vi "maintenance.vi"() -> ()   [LabVIEW 2019, in "Maintenance.lvlib"]
uses:
  Maintenance.lvlib
panel:
  out "String":string
  out "Tab Control":T1(tab)
  out "Query Verify":errorcluster
  out "Login Log":errorcluster
  out "Login Data Query":errorcluster
  out "General Setting Log":errorcluster
  out "General Setting Database":errorcluster
  out "Threshold Log":errorcluster
  out "Threshold Database":errorcluster
  out "Calibration Method 2 Table":errorcluster
  out "Calibration Method 2 Log":errorcluster
  out "Calibration Method 1 Table":errorcluster
  out "Calibration Method 1 Log":errorcluster
  out "Calibration Method 1 Database":errorcluster
  out "Calibration Setting Log":errorcluster
  out "Calibration Setting Table":errorcluster
  out "Start Application Log":errorcluster
  out "User Table":errorcluster
  out "Log Catalog Table":errorcluster
  out "Search in Log Table":errorcluster
  out "Search in Grading Tables":errorcluster
  out "Save to Excel Report":errorcluster
  out "Print Report":errorcluster
  out "Live View Open VI":errorcluster
  out "Setting Open VI":errorcluster
  out "Report Open VI":errorcluster
  out "Maintenance Open VI":errorcluster
  out "Login Open VI":errorcluster
  out "Logout Log":errorcluster
  out "Graphes Open VI":errorcluster
  out "Shutdown Application Log":errorcluster
  out "Restart Application Log":errorcluster
  out "Close Application Log":errorcluster
  out "Python Close Session":errorcluster
  out "Python Open Session":errorcluster
  out "Python Session out Disc 26":errorcluster
  out "IMAQdx Grab Disc 26":errorcluster
  out "Proc. Calibration Database Disc 26":errorcluster
  out "Python Session in Disc 26":errorcluster
  out "Processing Calibration Disc 26":errorcluster
  out "Speed Signal Log Disc 26":errorcluster
  out "Threshold Calibration Log Disc 26":errorcluster
  out "Main Grading Database Disc 26":errorcluster
  out "Grading Database Disc 26":errorcluster
  out "Pixel to mm Disc 26":errorcluster
  out "Draw Circule Disc 26":errorcluster
  out "IMAQ Copy Disc 26":errorcluster
  out "Log 10001~40002 Disc 26":errorcluster
  out "Image in Disc 26":errorcluster
  out "Image out Disc 26":errorcluster
  out "Python Session out Disc 27":errorcluster
  out "IMAQdx Grab Disc 27":errorcluster
  out "Proc. Calibration Database Disc 27":errorcluster
  out "Python Session in Disc 27":errorcluster
  out "Processing Calibration Disc 27":errorcluster
  out "Speed Signal Log Disc 27":errorcluster
  out "Threshold Calibration Log Disc 27":errorcluster
  out "Main Grading Database Disc 27":errorcluster
  out "Grading Database Disc 27":errorcluster
  out "Pixel to mm Disc 27":errorcluster
  out "Draw Circule Disc 27":errorcluster
  out "IMAQ Copy Disc 27":errorcluster
  out "Image in Disc 27":errorcluster
  out "Image out Disc 27":errorcluster
  out "Log 10001~40002 Disc 27":errorcluster
  out "Python Session out Disc 28":errorcluster
  out "IMAQdx Grab Disc 28":errorcluster
  out "Proc. Calibration Database Disc 28":errorcluster
  out "Python Session in Disc 28":errorcluster
  out "Processing Calibration Disc 28":errorcluster
  out "Speed Signal Log Disc 28":errorcluster
  out "Threshold Calibration Log Disc 28":errorcluster
  out "Main Grading Database Disc 28":errorcluster
  out "Grading Database Disc 28":errorcluster
  out "Pixel to mm Disc 28":errorcluster
  out "Draw Circule Disc 28":errorcluster
  out "IMAQ Copy Disc 28":errorcluster
  out "Image in Disc 28":errorcluster
  out "Image out Disc 28":errorcluster
  out "Log 10001~40002 Disc 28":errorcluster
  out "Python Session out Disc 29":errorcluster
  out "IMAQdx Grab Disc 29":errorcluster
  out "Proc. Calibration Database Disc 29":errorcluster
  out "Python Session in Disc 29":errorcluster
  out "Processing Calibration Disc 29":errorcluster
  out "Speed Signal Log Disc 29":errorcluster
  out "Threshold Calibration Log Disc 29":errorcluster
  out "Main Grading Database Disc 29":errorcluster
  out "Grading Database Disc 29":errorcluster
  out "Pixel to mm Disc 29":errorcluster
  out "Draw Circule Disc 29":errorcluster
  out "IMAQ Copy Disc 29":errorcluster
  out "Image in Disc 29":errorcluster
  out "Image out Disc 29":errorcluster
  out "Log 10001~40002 Disc 29":errorcluster
  out "Python Session out Disc 30":errorcluster
  out "IMAQdx Grab Disc 30":errorcluster
  out "Proc. Calibration Database Disc 30":errorcluster
  out "Python Session in Disc 30":errorcluster
  out "Processing Calibration Disc 30":errorcluster
  out "Speed Signal Log Disc 30":errorcluster
  out "Threshold Calibration Log Disc 30":errorcluster
  out "Main Grading Database Disc 30":errorcluster
  out "Grading Database Disc 30":errorcluster
  out "Pixel to mm Disc 30":errorcluster
  out "Draw Circule Disc 30":errorcluster
  out "IMAQ Copy Disc 30":errorcluster
  out "Image in Disc 30":errorcluster
  out "Image out Disc 30":errorcluster
  out "Log 10001~40002 Disc 30":errorcluster
  in  "Close":bool
  in  "General":bool
  in  "Disc 30":bool
  in  "Disc 29":bool
  in  "Disc 28":bool
  in  "Disc 27":bool
  in  "Disc 26":bool
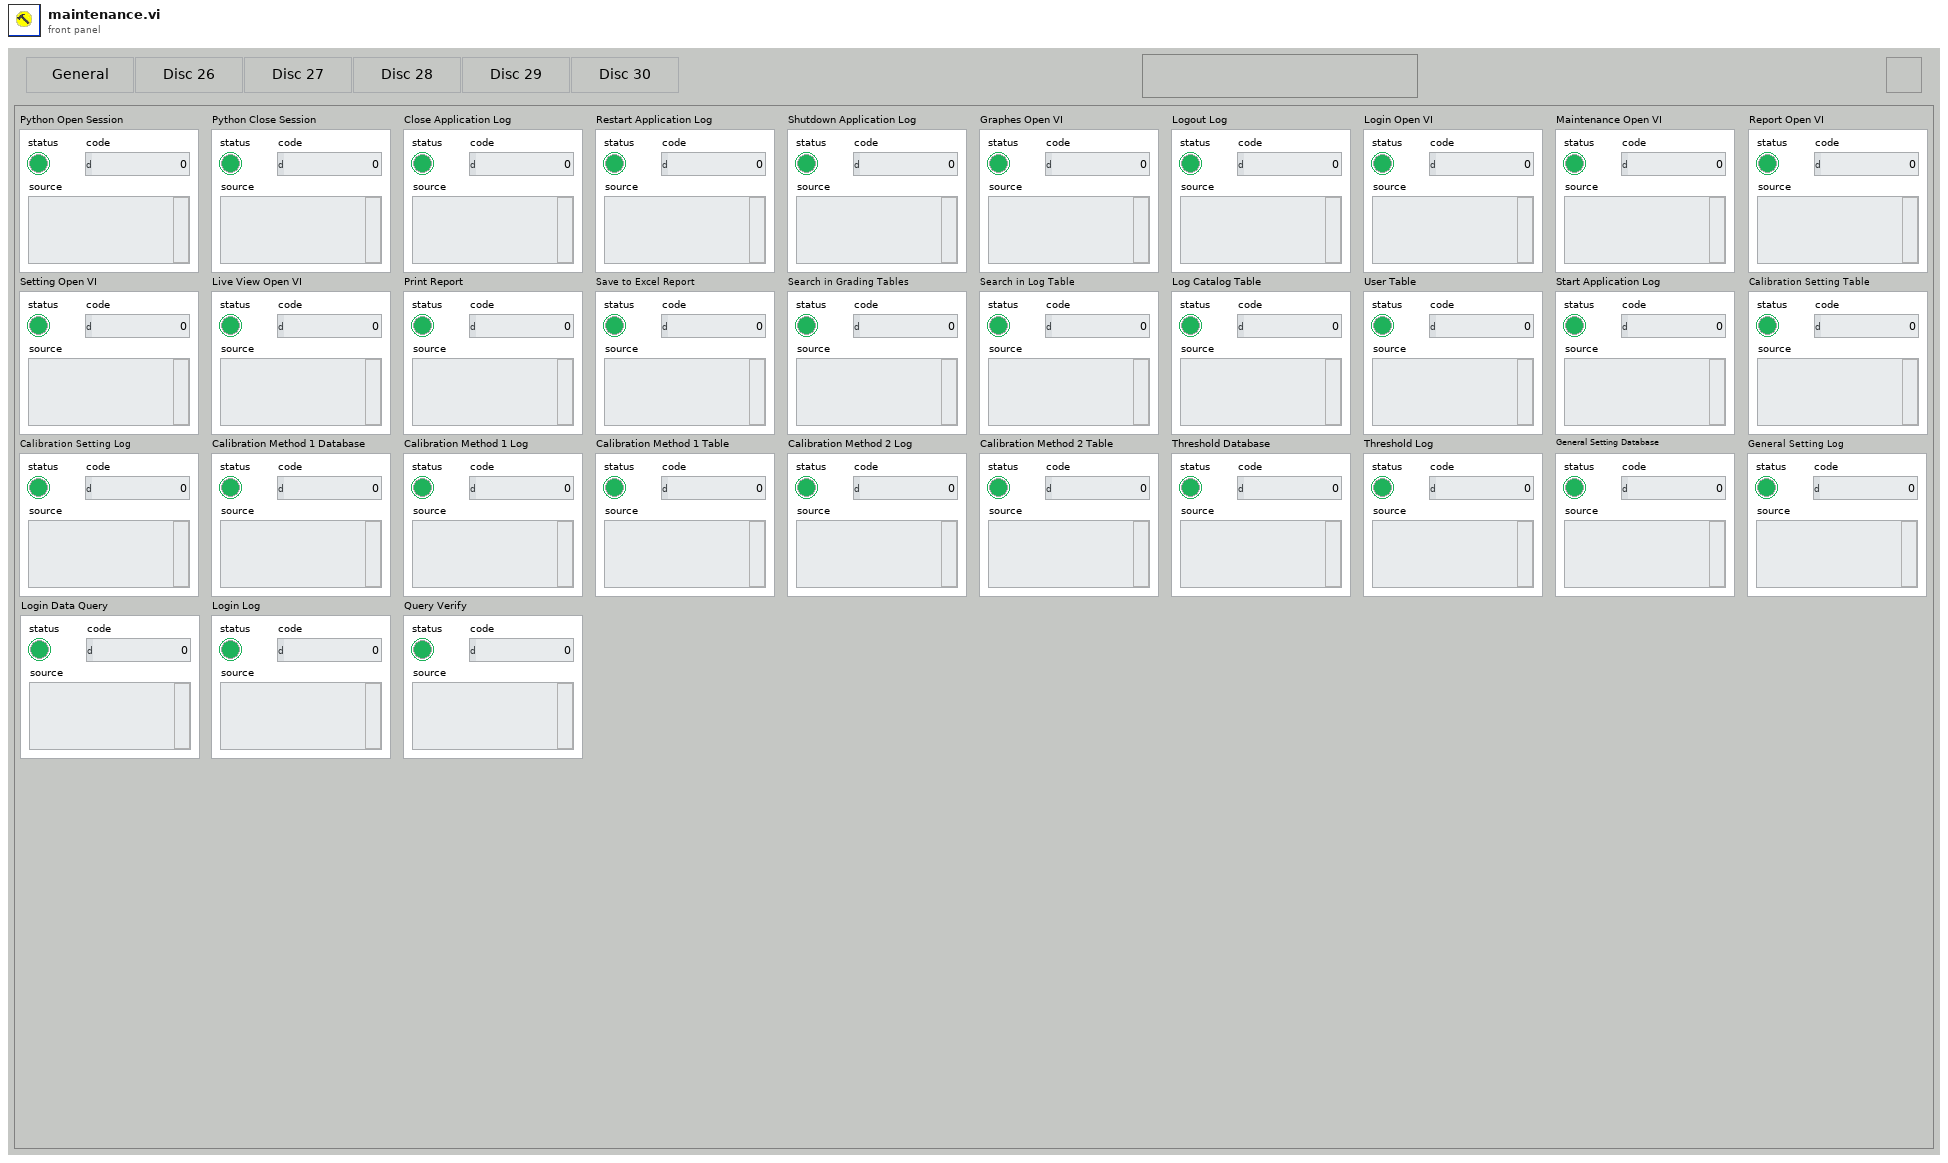
[diagram p1: front panel]
types:
  T1 = enum32{"General", "Disc 26", "Disc 27", "Disc 28", "Disc 29", "Disc 30"}
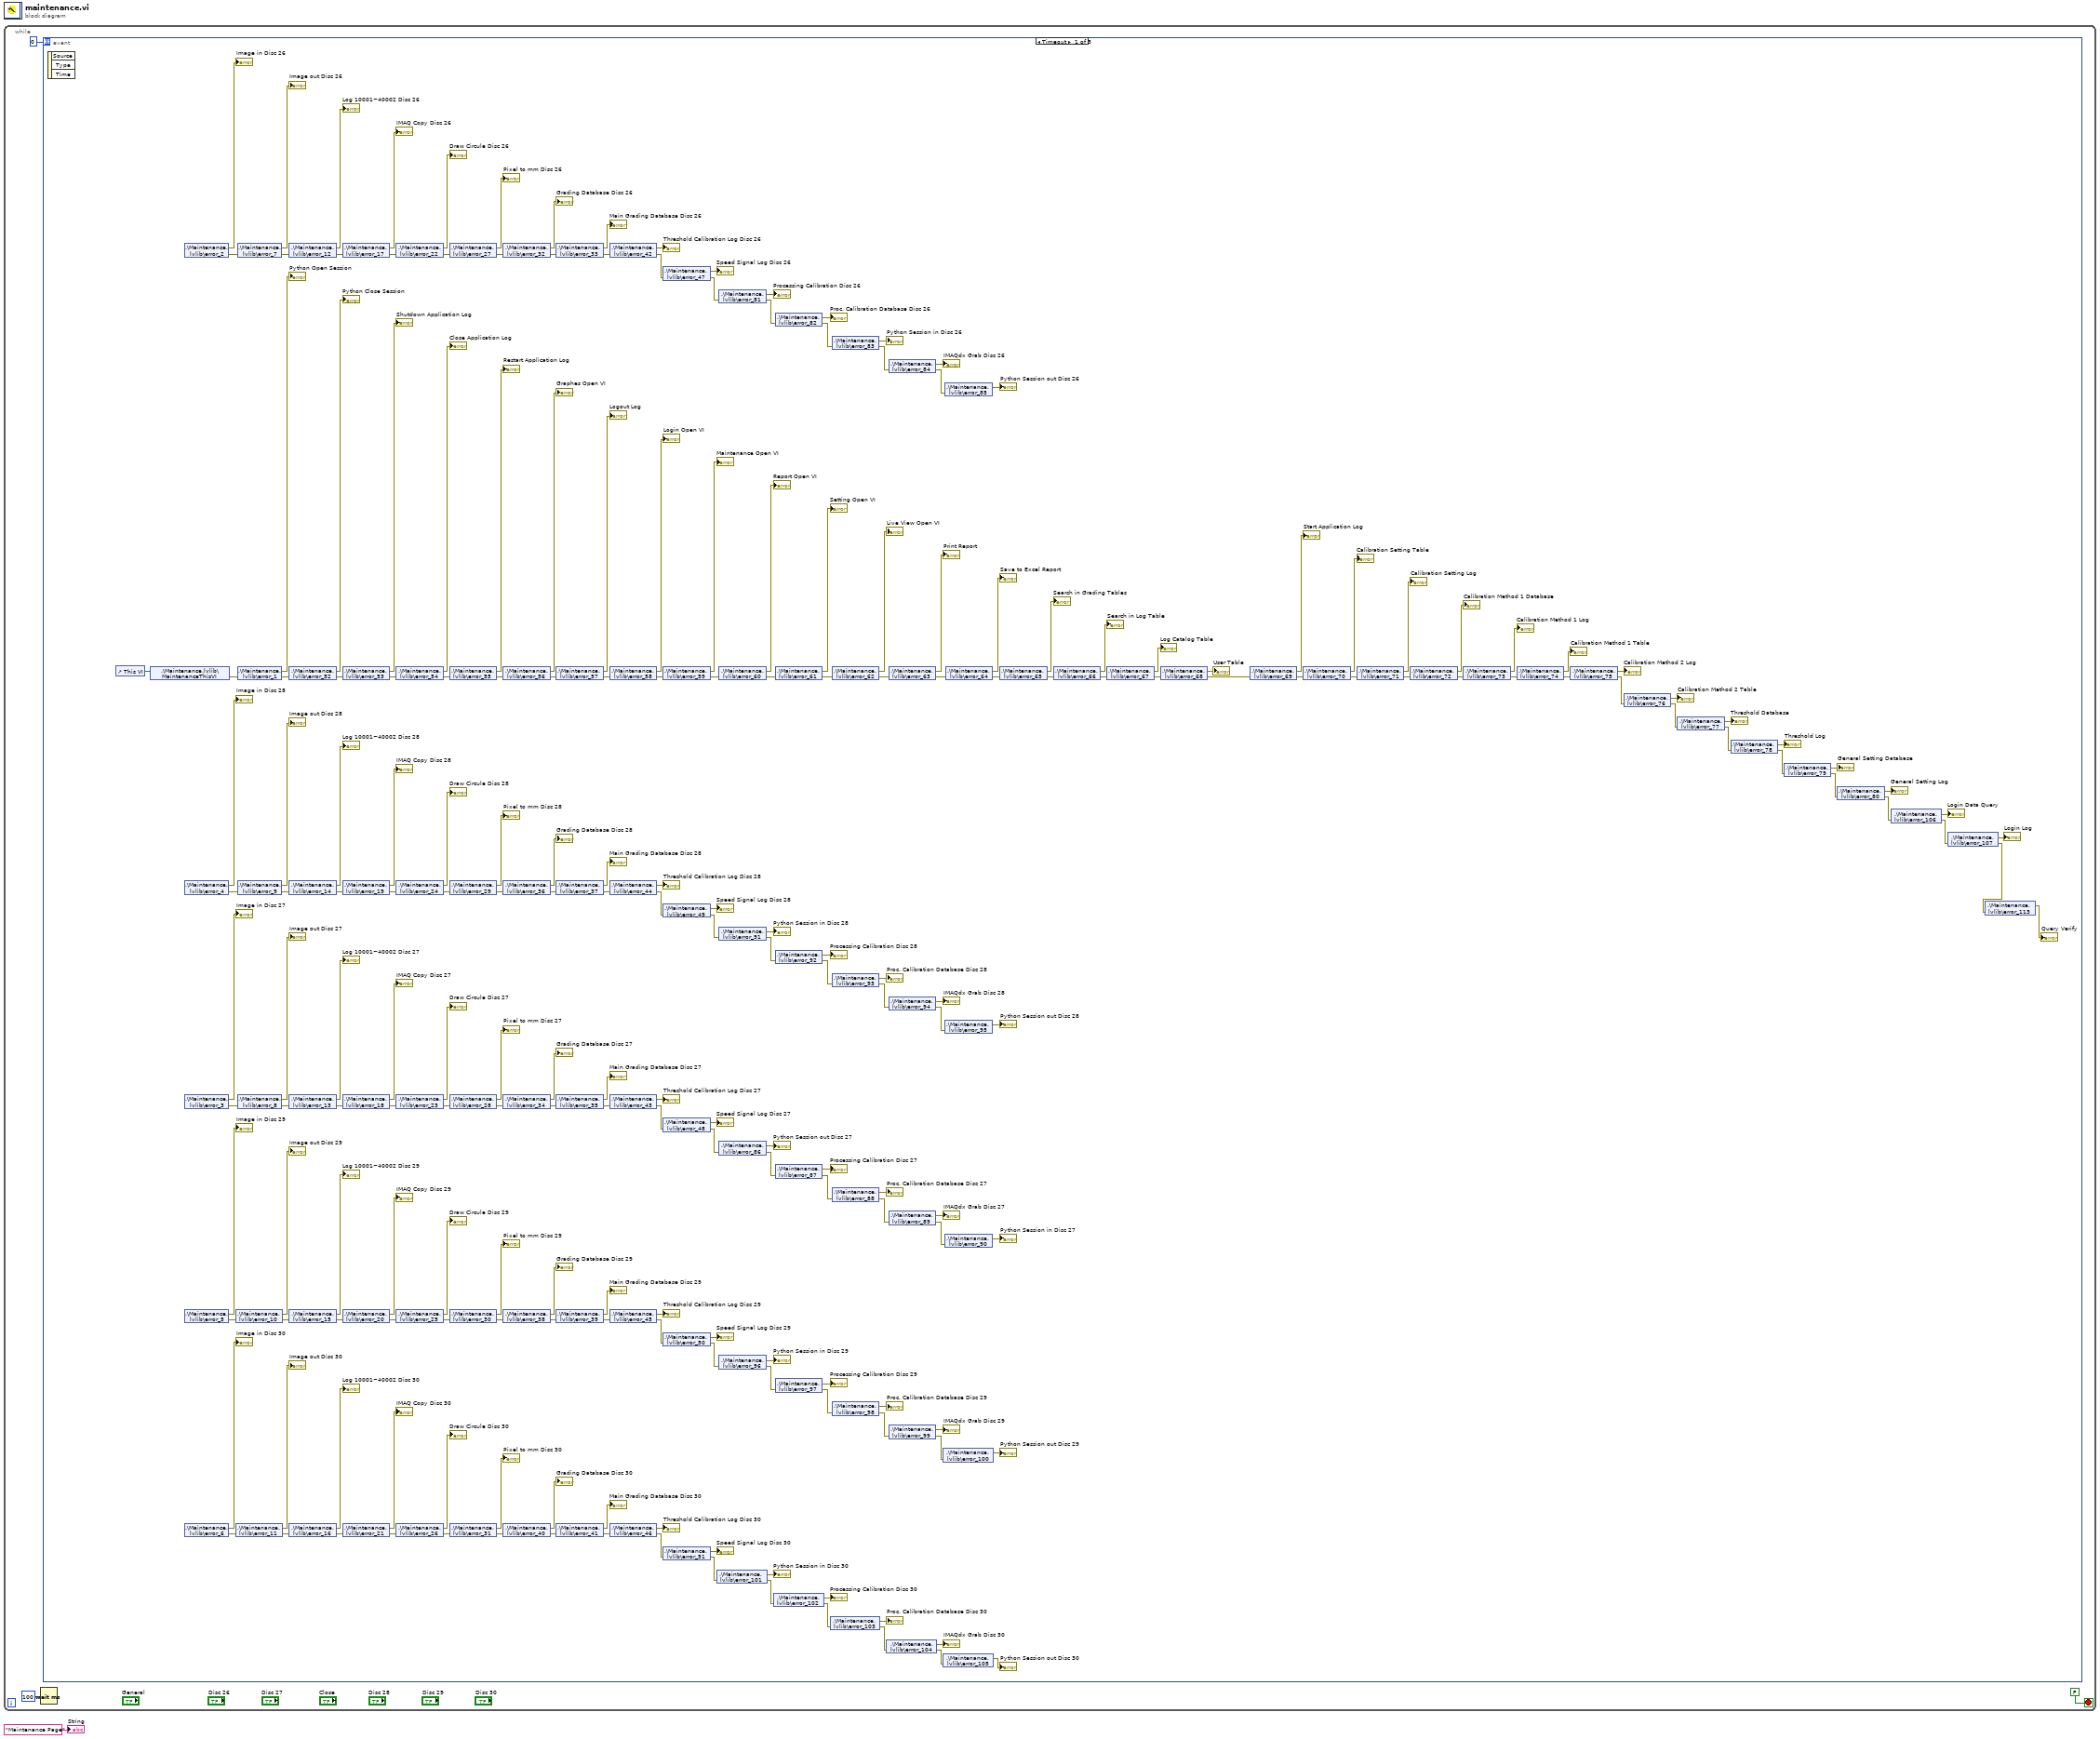
[diagram p0: block diagram]
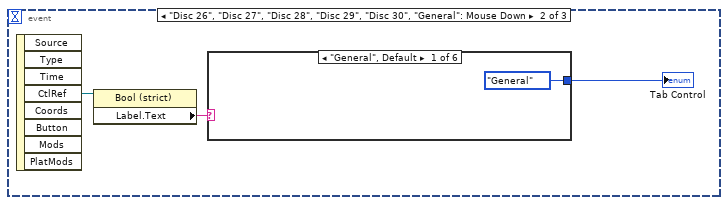
[diagram p2: hidden frame]
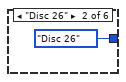
[diagram p3: hidden frame]
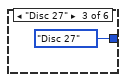
[diagram p4: hidden frame]
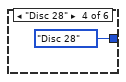
[diagram p5: hidden frame]
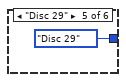
[diagram p6: hidden frame]
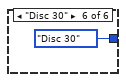
[diagram p7: hidden frame]
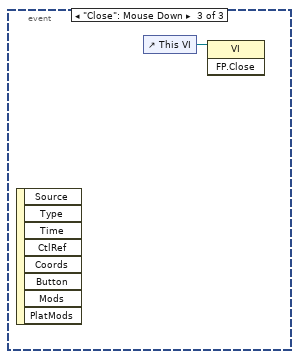
[diagram p8: hidden frame]
diagram:
  n1 = while {
    stop <- FALSE stop-if-true
    n2 = Wait (ms)(milliseconds to wait=u32 100) -> ()  [unwired: 1 out]
    n3 = event shown="[0] Timeout" {
      selector: _ -> [_ _ _]
      dyn-events: _ -> [_ _ _]
      timeout: 0 -> [_ _ _]
      event Timeout {
        n4 = event-data() -> ()  [unwired: 1 in, 3 out]
        n5 = control-ref of="This VI"() -> (w205:refnum<vi>)
        n6 = shared-variable ".\\Maintenance.lvlib\\MaintenanceThisVI"(w205) -> (error out=w189:errorcluster)  [unwired: 1 in]
        n7 = shared-variable ".\\Maintenance.lvlib\\error_2"() -> (→"Image in Disc 26":errorcluster, error out=w198:errorcluster)  [unwired: 1 in]
        n8 = shared-variable ".\\Maintenance.lvlib\\error_4"() -> (→"Image in Disc 28":errorcluster, error out=w199:errorcluster)  [unwired: 1 in]
        n9 = shared-variable ".\\Maintenance.lvlib\\error_3"() -> (→"Image in Disc 27":errorcluster, error out=w194:errorcluster)  [unwired: 1 in]
        n10 = shared-variable ".\\Maintenance.lvlib\\error_5"() -> (→"Image in Disc 29":errorcluster, error out=w195:errorcluster)  [unwired: 1 in]
        n11 = shared-variable ".\\Maintenance.lvlib\\error_6"() -> (→"Image in Disc 30":errorcluster, error out=w193:errorcluster)  [unwired: 1 in]
        n12 = shared-variable ".\\Maintenance.lvlib\\error_10"(error in=w195) -> (→"Image out Disc 29":errorcluster, error out=w190:errorcluster)
        n13 = shared-variable ".\\Maintenance.lvlib\\error_11"(error in=w193) -> (→"Image out Disc 30":errorcluster, error out=w192:errorcluster)
        n14 = shared-variable ".\\Maintenance.lvlib\\error_7"(error in=w198) -> (→"Image out Disc 26":errorcluster, error out=w197:errorcluster)
        n15 = shared-variable ".\\Maintenance.lvlib\\error_1"(error in=w189) -> (→"Python Open Session":errorcluster, error out=w127:errorcluster)
        n16 = shared-variable ".\\Maintenance.lvlib\\error_9"(error in=w199) -> (→"Image out Disc 28":errorcluster, error out=w196:errorcluster)
        n17 = shared-variable ".\\Maintenance.lvlib\\error_8"(error in=w194) -> (→"Image out Disc 27":errorcluster, error out=w191:errorcluster)
        n18 = shared-variable ".\\Maintenance.lvlib\\error_12"(error in=w197) -> (→"Log 10001~40002 Disc 26":errorcluster, error out=w187:errorcluster)
        n19 = shared-variable ".\\Maintenance.lvlib\\error_52"(error in=w127) -> (→"Python Close Session":errorcluster, error out=w111:errorcluster)
        n20 = shared-variable ".\\Maintenance.lvlib\\error_14"(error in=w196) -> (→"Log 10001~40002 Disc 28":errorcluster, error out=w184:errorcluster)
        n21 = shared-variable ".\\Maintenance.lvlib\\error_13"(error in=w191) -> (→"Log 10001~40002 Disc 27":errorcluster, error out=w185:errorcluster)
        n22 = shared-variable ".\\Maintenance.lvlib\\error_15"(error in=w190) -> (→"Log 10001~40002 Disc 29":errorcluster, error out=w181:errorcluster)
        n23 = shared-variable ".\\Maintenance.lvlib\\error_16"(error in=w192) -> (→"Log 10001~40002 Disc 30":errorcluster, error out=w179:errorcluster)
        n24 = shared-variable ".\\Maintenance.lvlib\\error_17"(error in=w187) -> (→"IMAQ Copy Disc 26":errorcluster, error out=w169:errorcluster)
        n25 = shared-variable ".\\Maintenance.lvlib\\error_53"(error in=w111) -> (→"Shutdown Application Log":errorcluster, error out=w113:errorcluster)
        n26 = shared-variable ".\\Maintenance.lvlib\\error_19"(error in=w184) -> (→"IMAQ Copy Disc 28":errorcluster, error out=w171:errorcluster)
        n27 = shared-variable ".\\Maintenance.lvlib\\error_18"(error in=w185) -> (→"IMAQ Copy Disc 27":errorcluster, error out=w175:errorcluster)
        n28 = shared-variable ".\\Maintenance.lvlib\\error_20"(error in=w181) -> (→"IMAQ Copy Disc 29":errorcluster, error out=w173:errorcluster)
        n29 = shared-variable ".\\Maintenance.lvlib\\error_21"(error in=w179) -> (→"IMAQ Copy Disc 30":errorcluster, error out=w177:errorcluster)
        n30 = shared-variable ".\\Maintenance.lvlib\\error_22"(error in=w169) -> (→"Draw Circule Disc 26":errorcluster, error out=w163:errorcluster)
        n31 = shared-variable ".\\Maintenance.lvlib\\error_54"(error in=w113) -> (→"Close Application Log":errorcluster, error out=w112:errorcluster)
        n32 = shared-variable ".\\Maintenance.lvlib\\error_24"(error in=w171) -> (→"Draw Circule Disc 28":errorcluster, error out=w161:errorcluster)
        n33 = shared-variable ".\\Maintenance.lvlib\\error_23"(error in=w175) -> (→"Draw Circule Disc 27":errorcluster, error out=w167:errorcluster)
        n34 = shared-variable ".\\Maintenance.lvlib\\error_25"(error in=w173) -> (→"Draw Circule Disc 29":errorcluster, error out=w159:errorcluster)
        n35 = shared-variable ".\\Maintenance.lvlib\\error_26"(error in=w177) -> (→"Draw Circule Disc 30":errorcluster, error out=w165:errorcluster)
        n36 = shared-variable ".\\Maintenance.lvlib\\error_27"(error in=w163) -> (→"Pixel to mm Disc 26":errorcluster, error out=w155:errorcluster)
        n37 = shared-variable ".\\Maintenance.lvlib\\error_55"(error in=w112) -> (→"Restart Application Log":errorcluster, error out=w110:errorcluster)
        n38 = shared-variable ".\\Maintenance.lvlib\\error_29"(error in=w161) -> (→"Pixel to mm Disc 28":errorcluster, error out=w147:errorcluster)
        n39 = shared-variable ".\\Maintenance.lvlib\\error_28"(error in=w167) -> (→"Pixel to mm Disc 27":errorcluster, error out=w152:errorcluster)
        n40 = shared-variable ".\\Maintenance.lvlib\\error_30"(error in=w159) -> (→"Pixel to mm Disc 29":errorcluster, error out=w143:errorcluster)
        n41 = shared-variable ".\\Maintenance.lvlib\\error_31"(error in=w165) -> (→"Pixel to mm Disc 30":errorcluster, error out=w139:errorcluster)
        n42 = shared-variable ".\\Maintenance.lvlib\\error_32"(error in=w155) -> (→"Grading Database Disc 26":errorcluster, error out=w158:errorcluster)
        n43 = shared-variable ".\\Maintenance.lvlib\\error_56"(error in=w110) -> (→"Graphes Open VI":errorcluster, error out=w108:errorcluster)
        n44 = shared-variable ".\\Maintenance.lvlib\\error_36"(error in=w147) -> (→"Grading Database Disc 28":errorcluster, error out=w150:errorcluster)
        n45 = shared-variable ".\\Maintenance.lvlib\\error_34"(error in=w152) -> (→"Grading Database Disc 27":errorcluster, error out=w151:errorcluster)
        n46 = shared-variable ".\\Maintenance.lvlib\\error_38"(error in=w143) -> (→"Grading Database Disc 29":errorcluster, error out=w146:errorcluster)
        n47 = shared-variable ".\\Maintenance.lvlib\\error_40"(error in=w139) -> (→"Grading Database Disc 30":errorcluster, error out=w142:errorcluster)
        n48 = shared-variable ".\\Maintenance.lvlib\\error_33"(error in=w158) -> (→"Main Grading Database Disc 26":errorcluster, error out=w138:errorcluster)
        n49 = shared-variable ".\\Maintenance.lvlib\\error_57"(error in=w108) -> (→"Logout Log":errorcluster, error out=w105:errorcluster)
        n50 = shared-variable ".\\Maintenance.lvlib\\error_37"(error in=w150) -> (→"Main Grading Database Disc 28":errorcluster, error out=w136:errorcluster)
        n51 = shared-variable ".\\Maintenance.lvlib\\error_35"(error in=w151) -> (→"Main Grading Database Disc 27":errorcluster, error out=w137:errorcluster)
        n52 = shared-variable ".\\Maintenance.lvlib\\error_39"(error in=w146) -> (→"Main Grading Database Disc 29":errorcluster, error out=w135:errorcluster)
        n53 = shared-variable ".\\Maintenance.lvlib\\error_41"(error in=w142) -> (→"Main Grading Database Disc 30":errorcluster, error out=w134:errorcluster)
        n54 = shared-variable ".\\Maintenance.lvlib\\error_42"(error in=w138) -> (→"Threshold Calibration Log Disc 26":errorcluster, error out=w119:errorcluster)
        n55 = shared-variable ".\\Maintenance.lvlib\\error_58"(error in=w105) -> (→"Login Open VI":errorcluster, error out=w103:errorcluster)
        n56 = shared-variable ".\\Maintenance.lvlib\\error_44"(error in=w136) -> (→"Threshold Calibration Log Disc 28":errorcluster, error out=w118:errorcluster)
        n57 = shared-variable ".\\Maintenance.lvlib\\error_43"(error in=w137) -> (→"Threshold Calibration Log Disc 27":errorcluster, error out=w120:errorcluster)
        n58 = shared-variable ".\\Maintenance.lvlib\\error_45"(error in=w135) -> (→"Threshold Calibration Log Disc 29":errorcluster, error out=w117:errorcluster)
        n59 = shared-variable ".\\Maintenance.lvlib\\error_46"(error in=w134) -> (→"Threshold Calibration Log Disc 30":errorcluster, error out=w121:errorcluster)
        n60 = shared-variable ".\\Maintenance.lvlib\\error_47"(error in=w119) -> (→"Speed Signal Log Disc 26":errorcluster, error out=w57:errorcluster)
        n61 = shared-variable ".\\Maintenance.lvlib\\error_59"(error in=w103) -> (→"Maintenance Open VI":errorcluster, error out=w101:errorcluster)
        n62 = shared-variable ".\\Maintenance.lvlib\\error_49"(error in=w118) -> (→"Speed Signal Log Disc 28":errorcluster, error out=w21:errorcluster)
        n63 = shared-variable ".\\Maintenance.lvlib\\error_48"(error in=w120) -> (→"Speed Signal Log Disc 27":errorcluster, error out=w41:errorcluster)
        n64 = shared-variable ".\\Maintenance.lvlib\\error_50"(error in=w117) -> (→"Speed Signal Log Disc 29":errorcluster, error out=w26:errorcluster)
        n65 = shared-variable ".\\Maintenance.lvlib\\error_51"(error in=w121) -> (→"Speed Signal Log Disc 30":errorcluster, error out=w11:errorcluster)
        n66 = shared-variable ".\\Maintenance.lvlib\\error_101"(error in=w11) -> (→"Python Session in Disc 30":errorcluster, error out=w20:errorcluster)
        n67 = shared-variable ".\\Maintenance.lvlib\\error_81"(error in=w57) -> (→"Processing Calibration Disc 26":errorcluster, error out=w60:errorcluster)
        n68 = shared-variable ".\\Maintenance.lvlib\\error_60"(error in=w101) -> (→"Report Open VI":errorcluster, error out=w100:errorcluster)
        n69 = shared-variable ".\\Maintenance.lvlib\\error_91"(error in=w21) -> (→"Python Session in Disc 28":errorcluster, error out=w40:errorcluster)
        n70 = shared-variable ".\\Maintenance.lvlib\\error_86"(error in=w41) -> (→"Python Session out Disc 27":errorcluster, error out=w47:errorcluster)
        n71 = shared-variable ".\\Maintenance.lvlib\\error_96"(error in=w26) -> (→"Python Session in Disc 29":errorcluster, error out=w25:errorcluster)
        n72 = shared-variable ".\\Maintenance.lvlib\\error_102"(error in=w20) -> (→"Processing Calibration Disc 30":errorcluster, error out=w19:errorcluster)
        n73 = shared-variable ".\\Maintenance.lvlib\\error_82"(error in=w60) -> (→"Proc. Calibration Database Disc 26":errorcluster, error out=w59:errorcluster)
        n74 = shared-variable ".\\Maintenance.lvlib\\error_61"(error in=w100) -> (→"Setting Open VI":errorcluster, error out=w97:errorcluster)
        n75 = shared-variable ".\\Maintenance.lvlib\\error_92"(error in=w40) -> (→"Processing Calibration Disc 28":errorcluster, error out=w39:errorcluster)
        n76 = shared-variable ".\\Maintenance.lvlib\\error_87"(error in=w47) -> (→"Processing Calibration Disc 27":errorcluster, error out=w48:errorcluster)
        n77 = shared-variable ".\\Maintenance.lvlib\\error_97"(error in=w25) -> (→"Processing Calibration Disc 29":errorcluster, error out=w24:errorcluster)
        n78 = shared-variable ".\\Maintenance.lvlib\\error_103"(error in=w19) -> (→"Proc. Calibration Database Disc 30":errorcluster, error out=w18:errorcluster)
        n79 = shared-variable ".\\Maintenance.lvlib\\error_83"(error in=w59) -> (→"Python Session in Disc 26":errorcluster, error out=w58:errorcluster)
        n80 = shared-variable ".\\Maintenance.lvlib\\error_62"(error in=w97) -> (→"Live View Open VI":errorcluster, error out=w96:errorcluster)
        n81 = shared-variable ".\\Maintenance.lvlib\\error_93"(error in=w39) -> (→"Proc. Calibration Database Disc 28":errorcluster, error out=w38:errorcluster)
        n82 = shared-variable ".\\Maintenance.lvlib\\error_88"(error in=w48) -> (→"Proc. Calibration Database Disc 27":errorcluster, error out=w49:errorcluster)
        n83 = shared-variable ".\\Maintenance.lvlib\\error_98"(error in=w24) -> (→"Proc. Calibration Database Disc 29":errorcluster, error out=w23:errorcluster)
        n84 = shared-variable ".\\Maintenance.lvlib\\error_104"(error in=w18) -> (→"IMAQdx Grab Disc 30":errorcluster, error out=w17:errorcluster)
        n85 = shared-variable ".\\Maintenance.lvlib\\error_84"(error in=w58) -> (→"IMAQdx Grab Disc 26":errorcluster, error out=w52:errorcluster)
        n86 = shared-variable ".\\Maintenance.lvlib\\error_63"(error in=w96) -> (→"Print Report":errorcluster, error out=w93:errorcluster)
        n87 = shared-variable ".\\Maintenance.lvlib\\error_94"(error in=w38) -> (→"IMAQdx Grab Disc 28":errorcluster, error out=w37:errorcluster)
        n88 = shared-variable ".\\Maintenance.lvlib\\error_89"(error in=w49) -> (→"IMAQdx Grab Disc 27":errorcluster, error out=w50:errorcluster)
        n89 = shared-variable ".\\Maintenance.lvlib\\error_99"(error in=w23) -> (→"IMAQdx Grab Disc 29":errorcluster, error out=w22:errorcluster)
        n90 = shared-variable ".\\Maintenance.lvlib\\error_100"(error in=w22) -> (→"Python Session out Disc 29":errorcluster)  [unwired: 1 out]
        n91 = shared-variable ".\\Maintenance.lvlib\\error_105"(error in=w17) -> (→"Python Session out Disc 30":errorcluster)  [unwired: 1 out]
        n92 = shared-variable ".\\Maintenance.lvlib\\error_85"(error in=w52) -> (→"Python Session out Disc 26":errorcluster)  [unwired: 1 out]
        n93 = shared-variable ".\\Maintenance.lvlib\\error_95"(error in=w37) -> (→"Python Session out Disc 28":errorcluster)  [unwired: 1 out]
        n94 = shared-variable ".\\Maintenance.lvlib\\error_90"(error in=w50) -> (→"Python Session in Disc 27":errorcluster)  [unwired: 1 out]
        n95 = shared-variable ".\\Maintenance.lvlib\\error_64"(error in=w93) -> (→"Save to Excel Report":errorcluster, error out=w91:errorcluster)
        n96 = shared-variable ".\\Maintenance.lvlib\\error_65"(error in=w91) -> (→"Search in Grading Tables":errorcluster, error out=w89:errorcluster)
        n97 = shared-variable ".\\Maintenance.lvlib\\error_66"(error in=w89) -> (→"Search in Log Table":errorcluster, error out=w88:errorcluster)
        n98 = shared-variable ".\\Maintenance.lvlib\\error_67"(error in=w88) -> (→"Log Catalog Table":errorcluster, error out=w87:errorcluster)
        n99 = shared-variable ".\\Maintenance.lvlib\\error_68"(error in=w87) -> (→"User Table":errorcluster, error out=w83:errorcluster)
        n100 = shared-variable ".\\Maintenance.lvlib\\error_69"(error in=w83) -> (→"Start Application Log":errorcluster, error out=w81:errorcluster)
        n101 = shared-variable ".\\Maintenance.lvlib\\error_70"(error in=w81) -> (→"Calibration Setting Table":errorcluster, error out=w80:errorcluster)
        n102 = shared-variable ".\\Maintenance.lvlib\\error_71"(error in=w80) -> (→"Calibration Setting Log":errorcluster, error out=w77:errorcluster)
        n103 = shared-variable ".\\Maintenance.lvlib\\error_72"(error in=w77) -> (→"Calibration Method 1 Database":errorcluster, error out=w78:errorcluster)
        n104 = shared-variable ".\\Maintenance.lvlib\\error_73"(error in=w78) -> (→"Calibration Method 1 Log":errorcluster, error out=w73:errorcluster)
        n105 = shared-variable ".\\Maintenance.lvlib\\error_74"(error in=w73) -> (→"Calibration Method 1 Table":errorcluster, error out=w72:errorcluster)
        n106 = shared-variable ".\\Maintenance.lvlib\\error_75"(error in=w72) -> (→"Calibration Method 2 Log":errorcluster, error out=w69:errorcluster)
        n107 = shared-variable ".\\Maintenance.lvlib\\error_76"(error in=w69) -> (→"Calibration Method 2 Table":errorcluster, error out=w67:errorcluster)
        n108 = shared-variable ".\\Maintenance.lvlib\\error_77"(error in=w67) -> (→"Threshold Database":errorcluster, error out=w68:errorcluster)
        n109 = shared-variable ".\\Maintenance.lvlib\\error_78"(error in=w68) -> (→"Threshold Log":errorcluster, error out=w61:errorcluster)
        n110 = shared-variable ".\\Maintenance.lvlib\\error_79"(error in=w61) -> (→"General Setting Database":errorcluster, error out=w64:errorcluster)
        n111 = shared-variable ".\\Maintenance.lvlib\\error_80"(error in=w64) -> (→"General Setting Log":errorcluster, error out=w9:errorcluster)
        n112 = shared-variable ".\\Maintenance.lvlib\\error_106"(error in=w9) -> (→"Login Data Query":errorcluster, error out=w7:errorcluster)
        n113 = shared-variable ".\\Maintenance.lvlib\\error_107"(error in=w7) -> (→"Login Log":errorcluster, error out=w6:errorcluster)
        n114 = shared-variable ".\\Maintenance.lvlib\\error_113"(error in=w6) -> (→"Query Verify":errorcluster)  [unwired: 1 out]
      }
      event "Disc 26", "Disc 27", "Disc 28", "Disc 29", "Disc 30", "General": Mouse Down {
        n115 = event-data() -> ("CtlRef"=w219:refnum<vi>)  [unwired: 1 in, 7 out]
        n116 = property class="Bool (strict)"(reference=w219) -> ("Label.Text"=w218:string)  [unwired: 1 in, 2 out]
        n117 = case shown="\"General\", Default" w218 {
          tunnel: [T1."General" ("Tab Control") T1."Disc 26" ("Tab Control") T1."Disc 27" ("Tab Control") T1."Disc 28" ("Tab Control") T1."Disc 29" ("Tab Control") T1."Disc 30" ("Tab Control")] -> w217
          frame "General", Default {
          }
          frame "Disc 26" {
          }
          frame "Disc 27" {
          }
          frame "Disc 28" {
          }
          frame "Disc 29" {
          }
          frame "Disc 30" {
          }
        }
        "Tab Control" <- w217
      }
      event "Close": Mouse Down {
        n118 = event-data() -> ()  [unwired: 1 in, 8 out]
        n119 = control-ref of="This VI"() -> (w226:refnum<vi>)
        n120 = invoke class="VI" method="FP.Close"(reference=w226) -> ()  [unwired: 2 in, 3 out]
      }
    }
  }
  "String" <- "Maintenance Page" ("String")
